vi "Patrick-Lockin-MAIN.vi"() -> ()   [LabVIEW 2013]
panel:
  in  "milliseconds to wait":u32
  out "Waveforms":dbl[][](graph)
  in  "Cluster 2":T1={"1/f vs. Uniform "=1.0, "DC Drift Fraction"=0.0, "DC Drift Freq"=0.19999999999999996, "DC Offset"=0.0, "60Hz Amplitude"=0.001, "Gauss/Unif %"=0.5, "Sig Amp"=3.0, "Noise Amp"=0.001} {"Noise Amp" format="%.1p"; "Sig Amp" format="%.2p"; "Gauss/Unif %" min=0.0 max=1.0 step=0.05 format="%.2f"; "60Hz Amplitude" min=0.0 max=10.0 step=0.05 format="%.2p"; "DC Offset" min=-1.0 max=1.0 step=0.01 format="%.2f"; "DC Drift Freq" min=0.0 max=5.0 step=0.05 format="%.2f"; "DC Drift Fraction" format="%.2f"; "1/f vs. Uniform" min=0.0 max=50.0 step=0.5 format="%.1p"}
  in  "Cluster":T1={"1/f vs. Uniform "=1.0, "DC Drift Fraction"=0.0, "DC Drift Freq"=0.19999999999999996, "DC Offset"=0.0, "60Hz Amplitude"=0.001, "Gauss/Unif %"=0.5, "Sig Amp"=3.0, "Noise Amp"=0.001} {"Noise Amp" format="%.1p"; "Sig Amp" format="%.2p"; "Gauss/Unif %" min=0.0 max=1.0 step=0.05 format="%.2f"; "60Hz Amplitude" min=0.0 max=10.0 step=0.05 format="%.2p"; "DC Offset" min=-1.0 max=1.0 step=0.01 format="%.2f"; "DC Drift Freq" min=0.0 max=5.0 step=0.05 format="%.2f"; "DC Drift Fraction" format="%.2f"; "1/f vs. Uniform" min=0.0 max=50.0 step=0.5 format="%.1p"}
  out "Avg Voltage vs. Time":T2(graph)
  in  "stop":bool
  in  "Rolling Avg Parameters":T3={"Rolling Avg mode"=enum."No Averaging", "# of averages"=10} {"# of averages" min=1}
  in  "Cutoff Freq":dbl[unit]=0.9 format="%.2f"
  in  "Sampling Info":cluster{"Fs":dbl[unit], "#S":i32}={"Fs"=55872.0, "#S"=8192}
  in  "Filter Type":T4(ring)=enum."Chebyshev"
  in  "Ref Phase":dbl=-1.6 format="%.2f"
  in  "Ref Frequency":dbl[unit]=1122.0 min=0.0 max=10000.0 step=50.0
  in  "Ref Amplitude":dbl=0.25 min=0.0 max=0.3 step=0.05 format="%.2f"
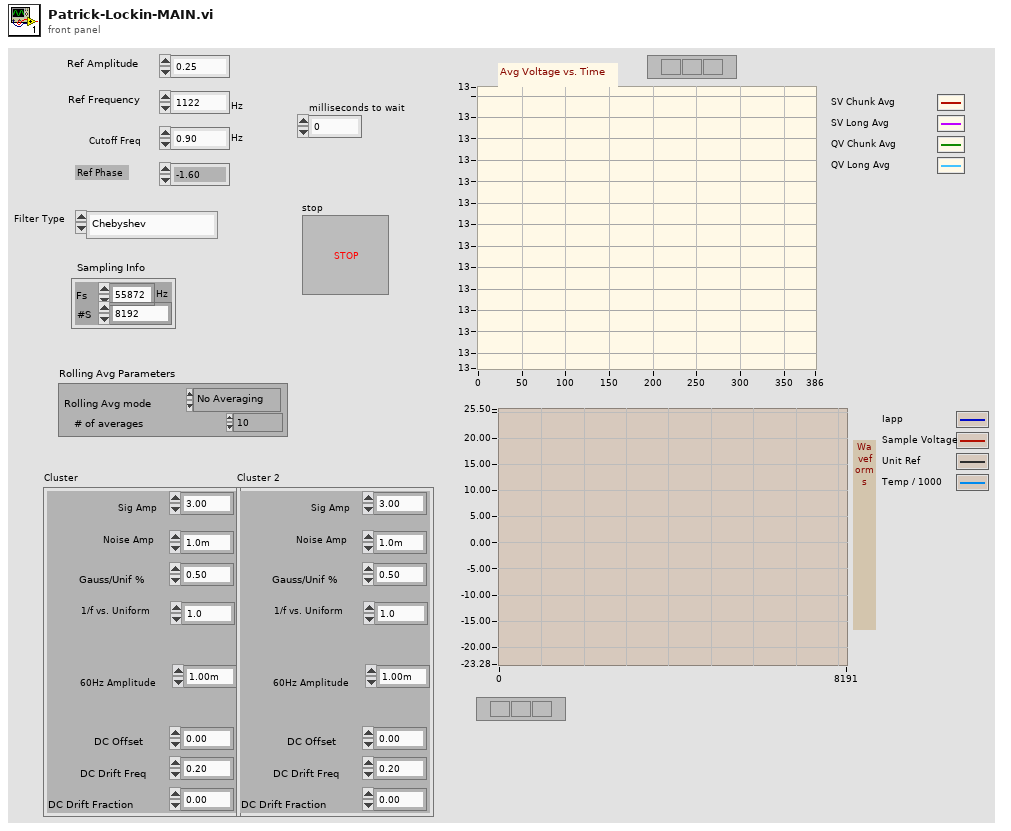
[diagram p1: front panel]
types:
  T1 = cluster{"1/f vs. Uniform ":dbl, "DC Drift Fraction":dbl, "DC Drift Freq":dbl, "DC Offset":dbl, "60Hz Amplitude":dbl, "Gauss/Unif %":dbl, "Sig Amp":dbl, "Noise Amp":dbl}
  T2 = cluster{"Chunk Average":dbl, "Chunk Average":dbl, "Chunk Average":dbl, "Chunk Average":dbl, "Long-term Average":dbl, "Long-term Average":dbl, "Long-term Average":dbl, "Long-term Average":dbl}
  T3 = cluster{"Rolling Avg mode":enum16{"No Averaging", "Linear", "Exponential"}, "# of averages":u32}
  T4 = enum16{"None", "Butterworth", "Chebyshev", "Inv Chebyshev"}
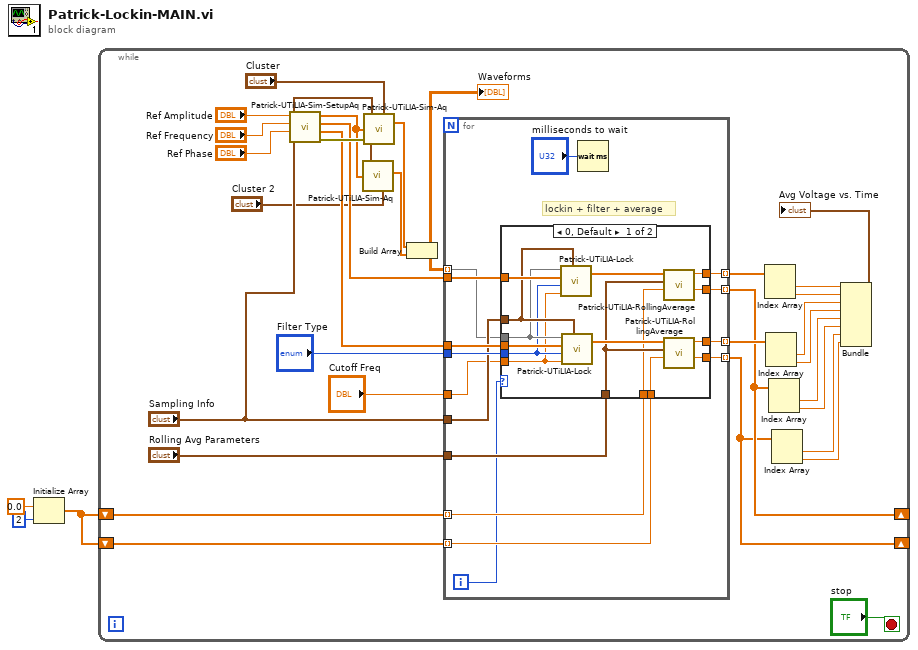
[diagram p0: block diagram]
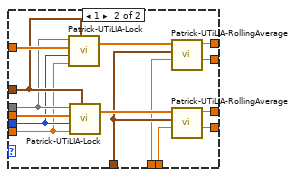
[diagram p2: hidden frame]
diagram:
  n1 = Initialize Array(0.0 ("element"), 2 ("dimension size")) -> (w1:dbl[])
  n2 = while {
    shift-right: [w8] -> _
    shift-left: w1 -> [w25]
    shift-right: [w9] -> _
    shift-left: w1 -> [w24]
    stop <- "stop" stop-if-true
    n3 = call "Patrick-UTiLIA-Sim-SetupAq.vi"("Sampling Info"="Sampling Info", "Ref Phase"="Ref Phase", "Ref Frequency"="Ref Frequency", "Ref Amplitude"="Ref Amplitude") -> ("Error out"=w32:errorcluster, "Unit Quadrature"=w30:dbl[], "Unit Reference"=w31:dbl[], "Scaled Reference"=w18:dbl[])  [unwired: 1 out]
    n4 = call "Patrick-UTiLIA-Sim-Aq.vi"("Cluster"="Cluster 2", "Sampling Info"="Sampling Info", "Scaled Reference"=w18) -> ("Sample Voltage"=w12:dbl[])  [unwired: 2 in, 2 out]
    n5 = call "Patrick-UTiLIA-Sim-Aq.vi"("Cluster"="Cluster", "Sampling Info"="Sampling Info", "Scaled Reference"=w18, "Error in"=w32) -> ("Sample Voltage"=w11:dbl[])  [unwired: 1 in, 2 out]
    n6 = Build Array(w11, w12) -> (w10:dbl[][])
    "Waveforms" <- w10
    n7 = for {
      tunnel: w31 -> [w50]
      tunnel: w30 -> [w49]
      tunnel: "Filter Type" -> [w48]
      tunnel: "Sampling Info" -> [w47]
      tunnel: "Cutoff Freq" -> [w46]
      tunnel: "Rolling Avg Parameters" -> [w45]
      tunnel: [w44] -> w8 mode=indexing
      tunnel: [w43] -> w9 mode=indexing
      tunnel: w25 -> [w42] mode=indexing
      tunnel: w24 -> [w41] mode=indexing
      tunnel: [w40] -> w23 mode=indexing
      tunnel: [w39] -> w15 mode=indexing
      tunnel: w10 -> [w38] mode=indexing
      i -> [w36]
      # "lockin + filter + average"
      n8 = case shown="0, Default" w36 {
        tunnel: w50 -> [w65 w80]
        tunnel: w49 -> [w64 w79]
        tunnel: w48 -> [w52 w67]
        tunnel: w47 -> [w54 w69]
        tunnel: w46 -> [w51 w66]
        tunnel: w45 -> [w61 w76]
        tunnel: [w60 w75] -> w44
        tunnel: [w59 w74] -> w43
        tunnel: w42 -> [w58 w73]
        tunnel: w41 -> [w57 w72]
        tunnel: [w56 w71] -> w40
        tunnel: [w55 w70] -> w39
        tunnel: w38 -> [w53 w68]
        frame 0, Default {
          n9 = call "Patrick-UTiLIA-Lock.vi"("Sampling Info"=w54, "Cutoff Freq"=w51, "Filter Type"=w52, "Unit Reference"=w65, "Noisy Signal"=w53) -> ("Locked Signal"=w63:dbl[])  [unwired: 1 in, 1 out]
          n10 = call "Patrick-UTiLIA-Lock.vi"("Sampling Info"=w54, "Cutoff Freq"=w51, "Filter Type"=w52, "Unit Reference"=w64, "Noisy Signal"=w53) -> ("Locked Signal"=w62:dbl[])  [unwired: 1 in, 1 out]
          n11 = call "Patrick-UTiLIA-RollingAverage.vi"("Current Average"=w57, "Rolling Avg Parameters"=w61, "Signal to Average"=w63) -> ("Long-term Average"=w59:dbl, "Chunk Average"=w56:dbl)  [unwired: 1 in, 3 out]
          n12 = call "Patrick-UTiLIA-RollingAverage.vi"("Current Average"=w58, "Rolling Avg Parameters"=w61, "Signal to Average"=w62) -> ("Long-term Average"=w60:dbl, "Chunk Average"=w55:dbl)  [unwired: 1 in, 3 out]
        }
        frame 1 {
          n13 = call "Patrick-UTiLIA-Lock.vi"("Sampling Info"=w69, "Cutoff Freq"=w66, "Filter Type"=w67, "Unit Reference"=w80, "Noisy Signal"=w68) -> ("Locked Signal"=w78:dbl[])  [unwired: 1 in, 1 out]
          n14 = call "Patrick-UTiLIA-Lock.vi"("Sampling Info"=w69, "Cutoff Freq"=w66, "Filter Type"=w67, "Unit Reference"=w79, "Noisy Signal"=w68) -> ("Locked Signal"=w77:dbl[])  [unwired: 1 in, 1 out]
          n15 = call "Patrick-UTiLIA-RollingAverage.vi"("Current Average"=w72, "Rolling Avg Parameters"=w76, "Signal to Average"=w78) -> ("Long-term Average"=w74:dbl, "Chunk Average"=w71:dbl)  [unwired: 1 in, 3 out]
          n16 = call "Patrick-UTiLIA-RollingAverage.vi"("Current Average"=w73, "Rolling Avg Parameters"=w76, "Signal to Average"=w77) -> ("Long-term Average"=w75:dbl, "Chunk Average"=w70:dbl)  [unwired: 1 in, 3 out]
        }
      }
      n17 = Wait (ms)(milliseconds to wait="milliseconds to wait") -> ()  [unwired: 1 out]
    }
    n18 = Index Array(array=w23) -> (element #1=w17:dbl, element #2=w16:dbl)  [unwired: 2 in]
    n19 = Index Array(array=w15) -> (element #1=w14:dbl, element #2=w13:dbl)  [unwired: 2 in]
    n20 = Index Array(array=w9) -> (element #1=w7:dbl, element #2=w6:dbl)  [unwired: 2 in]
    n21 = Index Array(array=w8) -> (element #1=w5:dbl, element #2=w4:dbl)  [unwired: 2 in]
    n22 = Bundle("Chunk Average"=w17, "Chunk Average"=w16, "Chunk Average"=w14, "Chunk Average"=w13, "Long-term Average"=w7, "Long-term Average"=w6, "Long-term Average"=w5, "Long-term Average"=w4) -> (→"Avg Voltage vs. Time":T2)  [unwired: 1 in]
  }
